vi "1-LogicFunctions.vi"() -> ()   [LabVIEW 2015]
panel:
  in  "Function Selector":enum16{"1", "2", "3"}(ring)
  in  "stop":bool
  out "Boolean":bool
  in  "x4":bool
  in  "x3":bool
  in  "x2":bool
  in  "x1":bool
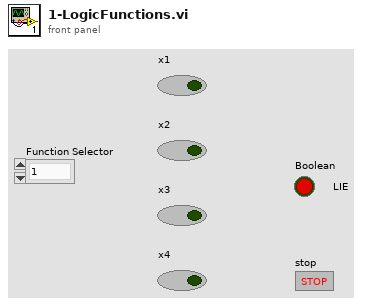
[diagram p1: front panel]
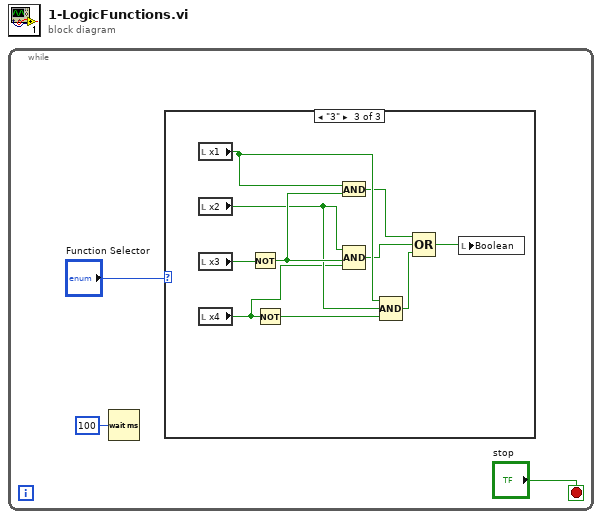
[diagram p0: block diagram]
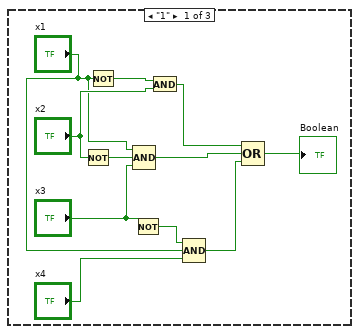
[diagram p2: hidden frame]
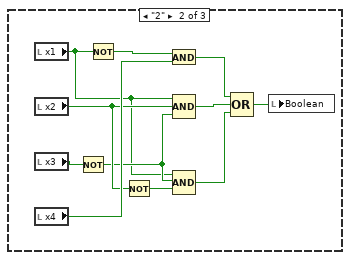
[diagram p3: hidden frame]
diagram:
  n1 = while {
    stop <- "stop" stop-if-true
    n2 = Wait (ms)(milliseconds to wait=u32 100) -> ()  [unwired: 1 out]
    n3 = case shown="\"3\"" "Function Selector" {
      frame "1" {
        n4 = Not(x="x2") -> (.not. x?=w14:bool)
        n5 = Not(x="x1") -> (.not. x?=w13:bool)
        n6 = Compound Arithmetic op=AND("x1", w14, "x3") -> (w10:bool)
        n7 = Not(x="x3") -> (.not. x?=w8:bool)
        n8 = And(x=w13, y="x2") -> (x .and. y?=w11:bool)
        n9 = Compound Arithmetic op=AND(w8, "x1", "x4") -> (w6:bool)
        n10 = Compound Arithmetic op=OR(w11, w10, w6) -> (→"Boolean":bool)
      }
      frame "2" {
        n11 = local read "x1"() -> (w19:bool)
        n12 = local read "x2"() -> (w22:bool)
        n13 = local read "x3"() -> (w23:bool)
        n14 = local read "x4"() -> (w25:bool)
        n15 = Not(x=w23) -> (.not. x?=w20:bool)
        n16 = Not(x=w19) -> (.not. x?=w24:bool)
        n17 = Not(x=w22) -> (.not. x?=w21:bool)
        n18 = And(x=w24, y=w25) -> (x .and. y?=w18:bool)
        n19 = Compound Arithmetic op=AND(w19, w22, w20) -> (w15:bool)
        n20 = Compound Arithmetic op=AND(w19, w20, w21) -> (w17:bool)
        n21 = Compound Arithmetic op=OR(w18, w15, w17) -> (w16:bool)
        n22 = local write "Boolean"(w16) -> ()
      }
      frame "3" {
        n23 = local read "x1"() -> (w33:bool)
        n24 = local read "x2"() -> (w32:bool)
        n25 = local read "x3"() -> (w35:bool)
        n26 = local read "x4"() -> (w30:bool)
        n27 = Not(x=w35) -> (.not. x?=w34:bool)
        n28 = Not(x=w30) -> (.not. x?=w31:bool)
        n29 = And(x=w33, y=w34) -> (x .and. y?=w29:bool)
        n30 = Compound Arithmetic op=AND(w32, w34, w30) -> (w28:bool)
        n31 = Compound Arithmetic op=AND(w33, w32, w31) -> (w26:bool)
        n32 = Compound Arithmetic op=OR(w29, w28, w26) -> (w27:bool)
        n33 = local write "Boolean"(w27) -> ()
      }
    }
  }
